vi "Begin.vi"(8 "error in":errorcluster) -> (0 "error out":errorcluster)   [LabVIEW 2020]
doc: "Called before other user functions, this VI is expected to open initial I/O refnums, load in file data, and do all program initialization. Notice that the <B>error out</B> terminal is simply used for data flow. Wiring it to other structures or subVIs ensures that this VI runs first."
uses:
  <vilib>/Rock Robotics/WPI/Encoder/WPI_EncoderType.ctl
  <vilib>/Rock Robotics/SystemInterfaces/DIO/FPGA_DIOChannel.ctl
  <vilib>/Rock Robotics/WPI/ThirdParty/Phoenix-LabVIEW/CANCoder/Controls/CTRE_Phoenix_CANcoder_Configurables.ctl
  <vilib>/Rock Robotics/WPI/ThirdParty/Phoenix-LabVIEW/CANCoder/Controls/CTRE_Phoenix_CANcoder_SensorInitializationStrategy.ctl
  <vilib>/Rock Robotics/WPI/ThirdParty/Phoenix-LabVIEW/CANCoder/Controls/CTRE_Phoenix_CANcoder_AbsoluteSensorRange.ctl
  <vilib>/Rock Robotics/WPI/ThirdParty/Phoenix-LabVIEW/Motor Controller/Controls/CTRE_Phoenix_MotorControl_VelocityMeasurementPeriod.ctl
  <vilib>/Rock Robotics/WPI/ThirdParty/Phoenix-LabVIEW/CANCoder/Controls/CTRE_Phoenix_CANcoder_SensorTimeBase.ctl
  <vilib>/Rock Robotics/WPI/DriverStation/WPI_DriverStationRobotMode2.ctl
  <vilib>/Rock Robotics/WPI/Joystick/WPI_JoystickDeviceEnum.ctl
  <vilib>/Rock Robotics/WPI/ThirdParty/REV Robotics/REVLib/Typedef/Spark MAX Motor Type.ctl
  <vilib>/Rock Robotics/WPI/ThirdParty/REV Robotics/REVLib/Typedef/Spark MAX Idle Mode.ctl
  <vilib>/Rock Robotics/WPI/SafetyOutput/WPI_SafetyOutputConfigMenu.ctl
  <vilib>/Rock Robotics/WPI/Solenoid/WPI_SolenoidChannel.ctl
  <vilib>/Rock Robotics/SystemInterfaces/DIO/FPGA_DIOPWMChannel.ctl
  Robot Global Data.vi
  <vilib>/Rock Robotics/Network Tables/NT Write String Array.vi
  <vilib>/Rock Robotics/WPI/Switch/WPI_SwitchOpenLimit.vi
  <vilib>/Rock Robotics/WPI/RobotDrive/WPI_RobotDriveOpen4MotorWithExistingMotors.vi
  <vilib>/Rock Robotics/WPI/Counter/WPI_CounterDigitalInputToDigitalSource.vi
  <vilib>/Rock Robotics/WPI/Solenoid/WPI_SolenoidOpenDouble.vi
  <vilib>/Rock Robotics/WPI/ThirdParty/Phoenix-LabVIEW/CANCoder/Set/CTRE_Phoenix_CANcoder_SetPosition.vi
panel:
  in  "CANcoder Configurables":T1={"Sensor Initialization Strategy"=enum."Boot To Zero", "Absolute Sensor Range"=enum."Unsigned [0 to 360)", "Velocity Measurement Period"=100, "Velocity Measurement Window"=64, "Magnet Offset (Degrees)"=0.0, "Sensor Direction"=FALSE, "Sensor Coefficient"=0.087890625, "Unit String"="deg", "Sensor Time Base"=enum."PerMinute"} {"Velocity Measurement Period" items=["Period_1ms"=1, "Period_2ms"=2, "Period_5ms"=5, "Period_10ms"=10, "Period_20ms"=20, "Period_25ms"=25, "Period_50ms"=50, "Period_100ms"=100]; "Sensor Coefficient" format="%#_9g"}
  in  "A Channel 2":T6=enum."DIO 2"
  in  "B Channel 2":T6=enum."DIO 3"
  in  "Invert Direction 2":bool
  in  "Decoding Type 2":T7=enum."4x"
  in  "DistancePerCount (Deg) 2":dbl=2.0
  in  "Minimum Rate 2":dbl=20.0
  in  "Number Samples to Average 2":u8=1
  in  "A Channel":T6
  in  "B Channel":T6=enum."DIO 1"
  in  "Invert Direction":bool
  in  "Decoding Type":T7=enum."4x"
  in  "DistancePerCount (Deg)":dbl=2.0
  in  "Minimum Rate":dbl=20.0
  in  "Number Samples to Average":u8=1
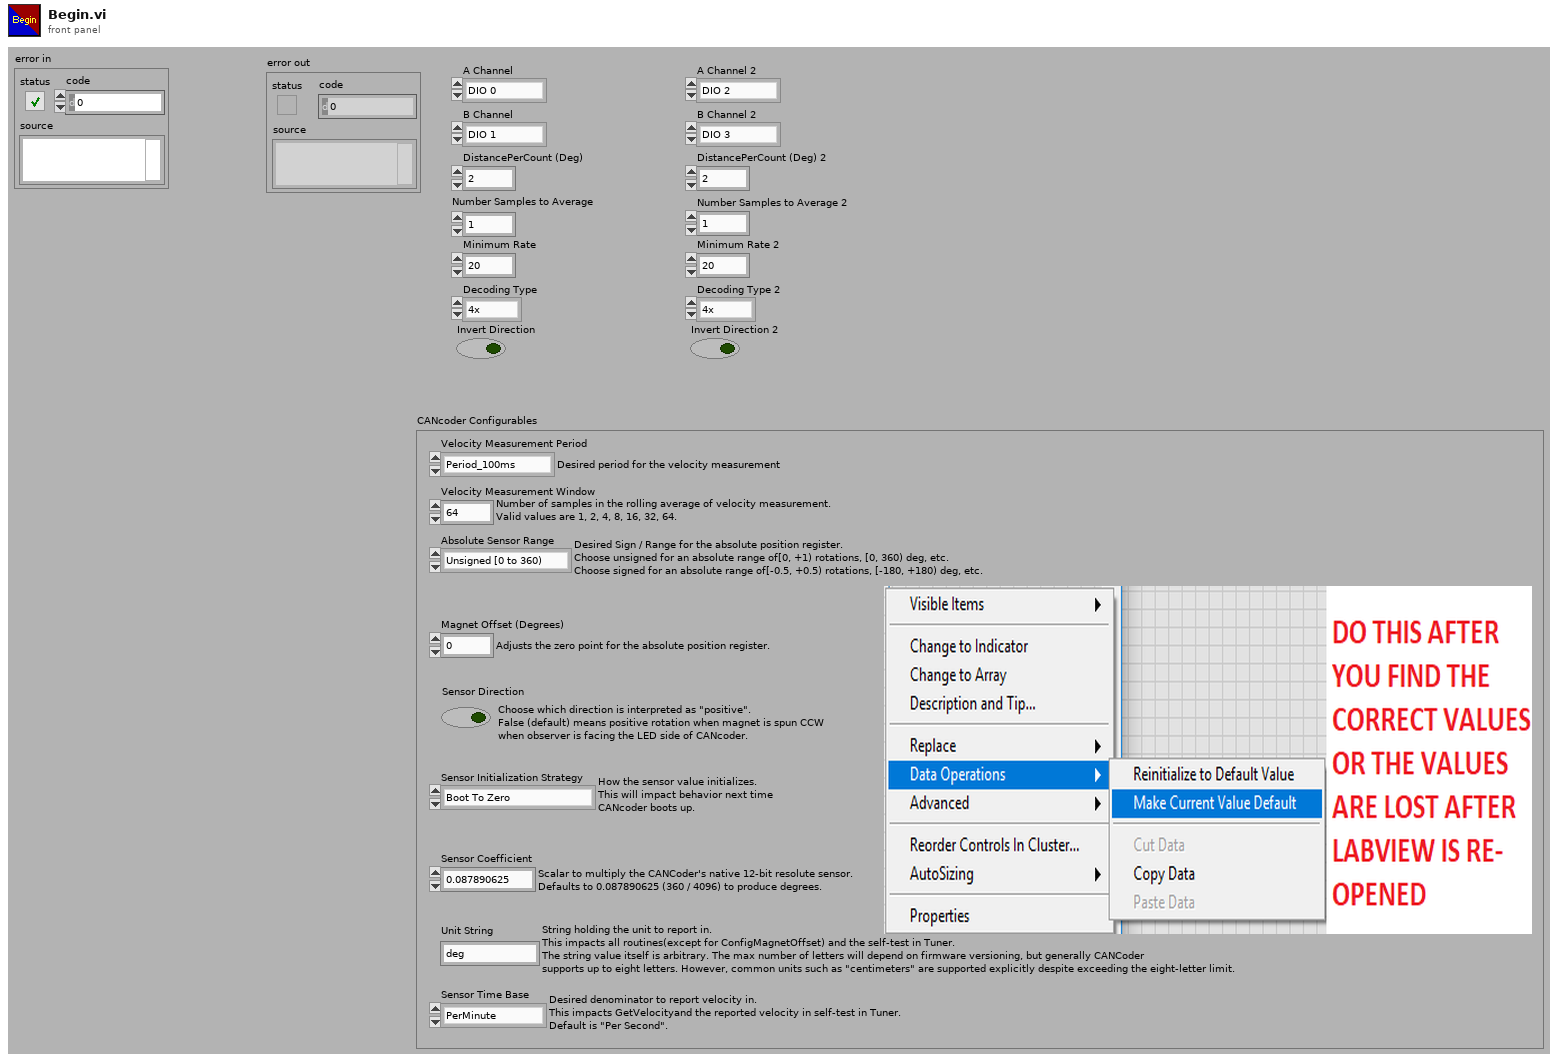
[diagram p1: front panel]
types:
  T1 = typedef "CTRE_Phoenix_CANcoder_Configurables.ctl" = cluster{"Sensor Initialization Strategy":T2, "Absolute Sensor Range":T3, "Velocity Measurement Period":T4, "Velocity Measurement Window":i32, "Magnet Offset (Degrees)":dbl, "Sensor Direction":bool, "Sensor Coefficient":dbl, "Unit String":string, "Sensor Time Base":T5}
  T2 = typedef "CTRE_Phoenix_CANcoder_SensorInitializationStrategy.ctl" = enum16{"Boot To Zero", "Boot To Absolute Position"}
  T3 = typedef "CTRE_Phoenix_CANcoder_AbsoluteSensorRange.ctl" = enum16{"Unsigned [0 to 360)", "Signed [-180 to +180)"}
  T4 = typedef "CTRE_Phoenix_MotorControl_VelocityMeasurementPeriod.ctl" = u16
  T5 = typedef "CTRE_Phoenix_CANcoder_SensorTimeBase.ctl" = enum16{"Per100Ms_Legacy", "PerSecond", "PerMinute"}
  T6 = typedef "FPGA_DIOChannel.ctl" = enum8{"DIO 0", "DIO 1", "DIO 2", "DIO 3", "DIO 4", "DIO 5", "DIO 6", "DIO 7", "DIO 8", "DIO 9", "DIO MXP 0", "DIO MXP 1", "DIO MXP 2", "DIO MXP 3", "DIO MXP 4", "DIO MXP 5", "DIO MXP 6", "DIO MXP 7", "DIO MXP 8", "DIO MXP 9", "DIO MXP 10", "DIO MXP 11", "DIO MXP 12", "DIO MXP 13", "DIO MXP 14", "DIO MXP 15", "SPI Port CS1", "SPI Port CS2", "SPI Port CS3", "SPI Port MISO", "SPI Port MOSI", "Invalid"}
  T7 = typedef "WPI_EncoderType.ctl" = enum16{"1x", "2x", "4x"}
  T8 = typedef "FPGA_DIOPWMChannel.ctl" = enum8{"PWM 0", "PWM 1", "PWM 2", "PWM 3", "PWM 4", "PWM 5", "PWM 6", "PWM 7", "PWM 8", "PWM 9", "PWM MXP 0", "PWM MXP 1", "PWM MXP 2", "PWM MXP 3", "PWM MXP 4", "PWM MXP 5", "PWM MXP 6", "PWM MXP 7", "PWM MXP 8", "PWM MXP 9", "Invalid"}
  T9 = typedef "WPI_SolenoidChannel.ctl" = enum8{"Solenoid 0", "Solenoid 1", "Solenoid 2", "Solenoid 3", "Solenoid 4", "Solenoid 5", "Solenoid 6", "Solenoid 7", "Solenoid 8", "Solenoid 9", "Solenoid 10", "Solenoid 11", "Solenoid 12", "Solenoid 13", "Solenoid 14", "Solenoid 15", "Invalid"}
  T10 = typedef "WPI_SafetyOutputConfigMenu.ctl" = enum16{"Enable", "Disable"}
  T11 = typedef "WPI_JoystickDeviceEnum.ctl" = enum16{"USB 0", "USB 1", "USB 2", "USB 3", "USB 4", "USB 5"}
  T12 = typedef "Spark MAX Idle Mode.ctl" = enum16{"Coast", "Brake"}
  T13 = typedef "Spark MAX Motor Type.ctl" = enum16{"Brushed", "Brushless"}
  T14 = typedef "WPI_DriverStationRobotMode2.ctl" = enum16{"Autonomous Disabled", "Autonomous Enabled", "Teleop Disabled", "Teleop Enabled", "Disconnected", "Finish", "Test Disabled", "Test Enabled", "Emergency Stopped"}
  T15 = typedef "WPI_MotorControlDeviceRef.ctl" = cluster{"DeviceStatus":errorcluster, "Type":T16, "PWM":cluster{"PWM Channel":T8, "DeadBand":T17}, "CAN":cluster{"Device Number":u8, "SetOutput VI Ref":variant, "GetOutput VI Ref":variant, "Enable VI Ref":variant, "Disable VI Ref":variant, "Data":variant}, "Invert":bool, "DIO PWM":cluster{"PWM \"Enable\" Channel":T8, "DIOChannel":T6, "PWM Rate":dbl}}
  T16 = typedef "WPI_MotorControlType.ctl" = enum16{"PWM", "CAN", "DIO PWM"}
  T17 = typedef "WPI_PWMDeadband.ctl" = cluster{"Name":string, "maxPositivePwm":i32, "minPositivePwm":i32, "centerPwm":i32, "maxNegativePwm":i32, "minNegativePwm":i32, "angularRange":u16}
  T18 = typedef "WPI_JoystickDevRef.ctl" = cluster{"Device":T11}
  T19 = typedef "WPI_RobotDriveDevRef.ctl" = cluster{"DevStatus":errorcluster, "Motors[]":T15[], "Square Inputs":bool, "Max Output":dbl}
  T20 = typedef "CTRE_Phoenix_CANcoder_DeviceRef.ctl" = cluster{"DeviceStatus":errorcluster, "Device Number":u8, "Handle":u64, "UsageFrame":u32, "Library Path":path}
  T21 = typedef "WPI_DigitalInputDevRef.ctl" = cluster{"DevStatus":errorcluster, "DIO Channel":T6}
  T22 = typedef "FPGA_CounterEncoderSourceConvertionLVSourceType.ctl" = cluster{"DevStatus":errorcluster, "AnalogTriggerMode?":bool, "DigitalMode":cluster{"DIO Channel":T23}, "AnalogTriggerMode":cluster{"AnalogTriggerIndex":T24, "OutputType":T25}}
  T23 = typedef "FPGA_DIODigitalSourceChannel.ctl" = enum8{"DIO 0", "DIO 1", "DIO 2", "DIO 3", "DIO 4", "DIO 5", "DIO 6", "DIO 7", "DIO 8", "DIO 9", "DIO MXP 0", "DIO MXP 1", "DIO MXP 2", "DIO MXP 3", "DIO MXP 4", "DIO MXP 5", "DIO MXP 6", "DIO MXP 7", "DIO MXP 8", "DIO MXP 9", "DIO MXP 10", "DIO MXP 11", "DIO MXP 12", "DIO MXP 13", "DIO MXP 14", "DIO MXP 15", "SPI Port CS1", "SPI Port CS2", "SPI Port CS3", "SPI Port MISO", "SPI Port MOSI", "Disabled"}
  T24 = typedef "FPGA_AnalogTriggerIndex.ctl" = enum8{"Trig 0", "Trig 1", "Trig 2", "Trig 3", "Trig 4", "Trig 5", "Trig 6", "Trig 7", "Invalid"}
  T25 = typedef "FPGA_AnalogTriggerOutType.ctl" = enum16{"InWindow", "TriggerState", "Rising", "Falling"}
  T26 = typedef "WPI_ServoDeviceRef.ctl" = cluster{"DeviceStatus":errorcluster, "PWM Channel":T8, "DeadBand":T17}
  T27 = typedef "WPI_EncoderDevRef.ctl" = cluster{"DevStatus":errorcluster, "EncoderIndex":T28, "CounterIndex":T29, "DistancePerCount":dbl, "Decoding Type":T7}
  T28 = typedef "FPGA_EncoderIdx.ctl" = enum8{"Enc 0", "Enc 1", "Enc 2", "Enc 3", "Enc 4", "Enc 5", "Enc 6", "Enc 7", "Invalid"}
  T29 = typedef "FPGA_CounterCtrSystemIndex.ctl" = enum8{"Ctr 0", "Ctr 1", "Ctr 2", "Ctr 3", "Ctr 4", "Ctr 5", "Ctr 6", "Ctr 7", "Invalid"}
  T30 = typedef "WPI_SwitchDevRef.ctl" = cluster{"DevStatus":errorcluster, "DIO Channel":T6, "CntIndex":T29, "Normally Closed":bool}
  T31 = typedef "WPI_SolenoidDevRef.ctl" = cluster{"DevStatus":errorcluster, "Pneumatics Control Module":u8, "Forward Solenoid Channel":T9, "Reverse Solenoid Channel":T9}
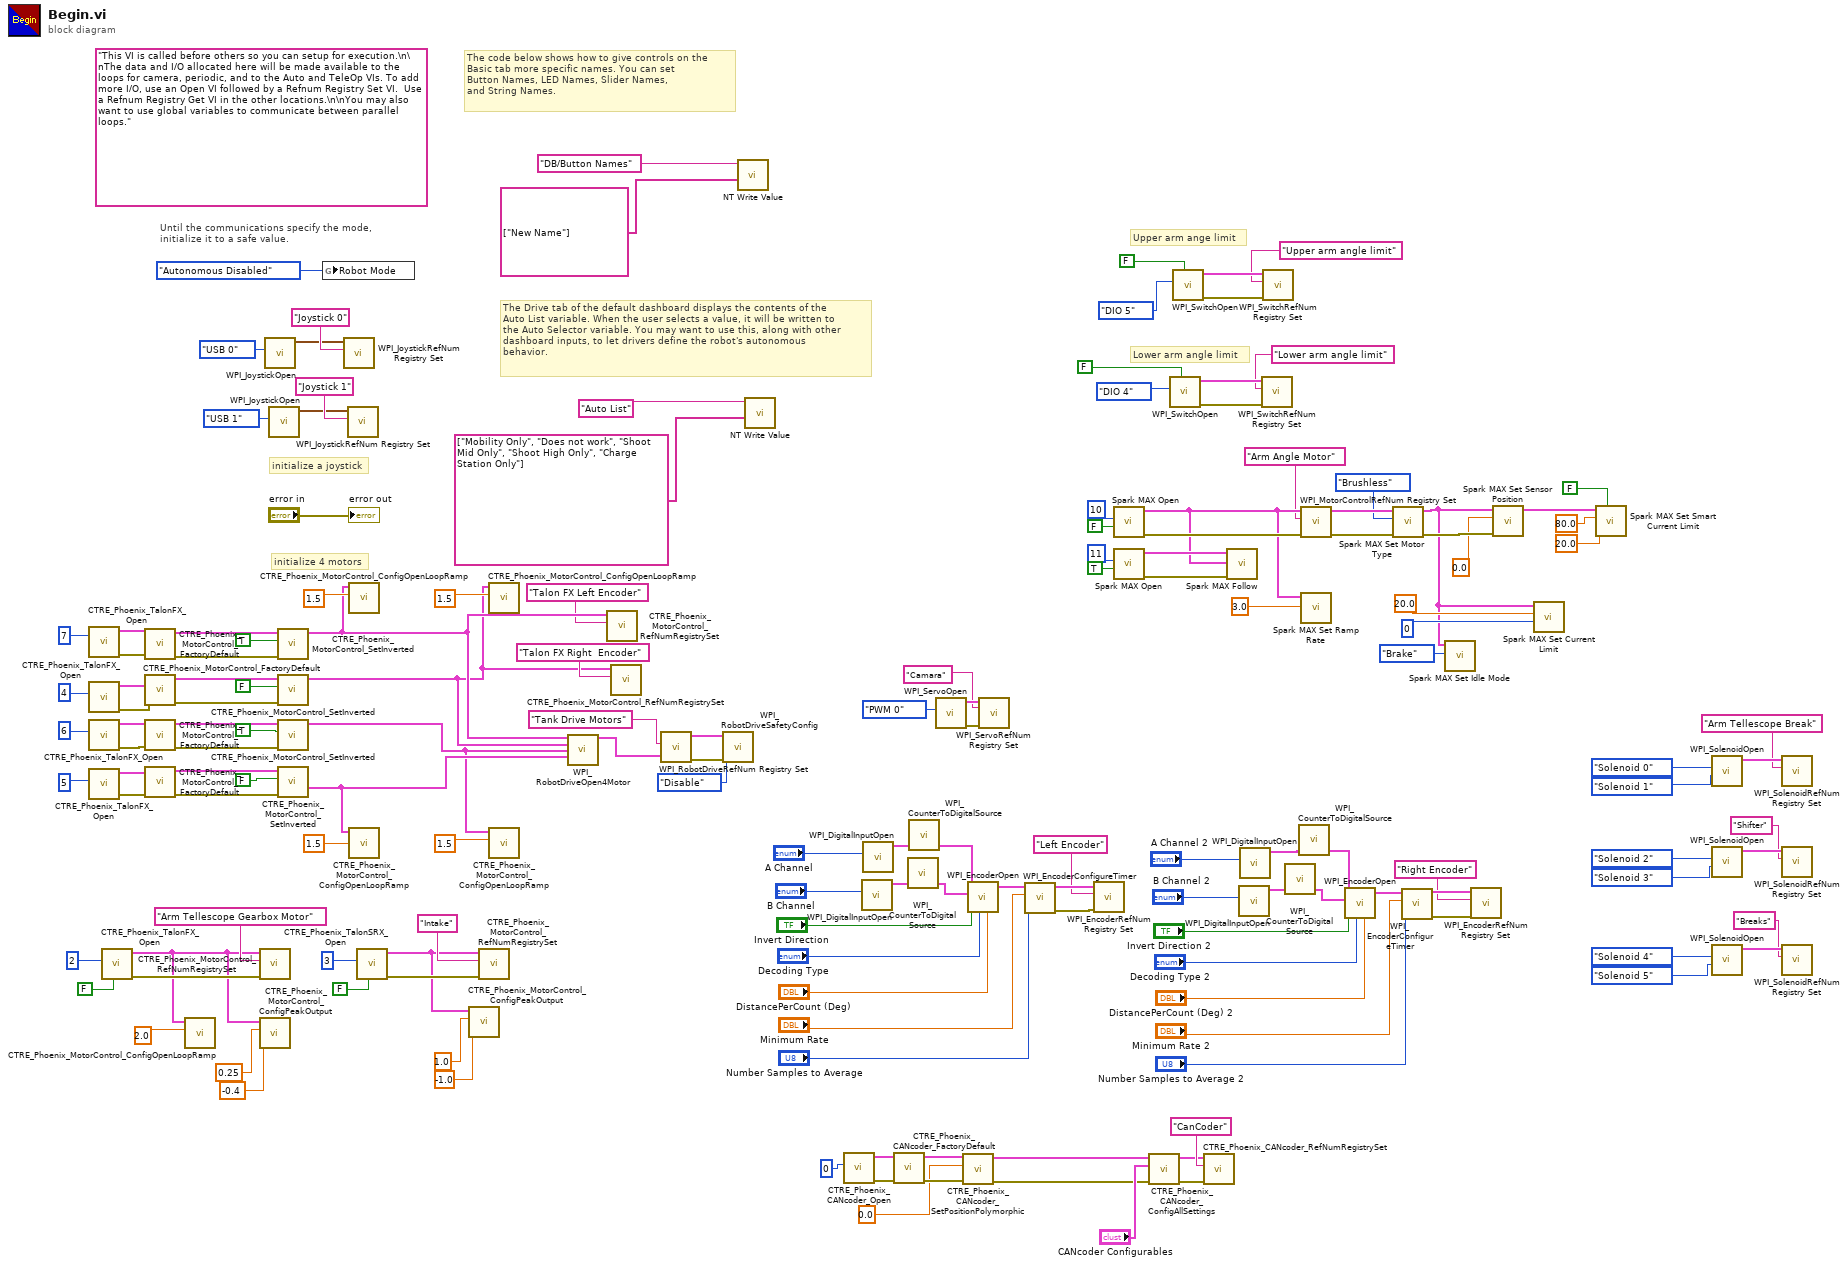
[diagram p0: block diagram]
diagram:
  (unwired) "This VI is called before others so you can setup for execution.\n\nThe data and I/O allocated here will be made available to the loops for camera, periodic, and to the Auto and TeleOp VIs. To add more I/O, use an Open VI followed by a Refnum Registry Set VI.  Use a Refnum Registry Get VI in the other locations.\n\nYou may also want to use global variables to communicate between parallel loops."
  # "Lower arm angle limit"
  # "Upper arm ange limit"
  # "The Drive tab of the default dashboard displays the contents of the\nAuto List variable. When the user selects a value, it will be written to\nthe Auto Selector variable. You may want to use this, along with other\ndashboard inputs, to let drivers define the robot's autonomous\nbehavior."
  # "The code below shows how to give controls on the\nBasic tab more specific names. You can set\nButton Names, LED Names, Slider Names,\nand String Names."
  # "initialize a joystick"
  # "Until the communications specify the mode,\ninitialize it to a safe value."
  # "initialize 4 motors"
  n1 = call <vilib>:"CTRE_Phoenix_TalonFX_Open.vi"("Device Number"=u8 7) -> ("error out"=w92:errorcluster, "PhoenixMotorControlDevRef"=w90:T15)  [unwired: 9 in]
  n2 = call <vilib>:"CTRE_Phoenix_TalonFX_Open.vi"("Device Number"=u8 4) -> ("error out"=w94:errorcluster, "PhoenixMotorControlDevRef"=w95:T15)  [unwired: 9 in]
  n3 = call <vilib>:"CTRE_Phoenix_TalonFX_Open.vi"("Device Number"=u8 6) -> ("error out"=w98:errorcluster, "PhoenixMotorControlDevRef"=w99:T15)  [unwired: 9 in]
  n4 = call <vilib>:"CTRE_Phoenix_TalonFX_Open.vi"("Device Number"=u8 5) -> ("error out"=w80:errorcluster, "PhoenixMotorControlDevRef"=w100:T15)  [unwired: 9 in]
  n5 = call <vilib>:"CTRE_Phoenix_TalonFX_Open.vi"("Invert"=FALSE, "Device Number"=u8 2) -> ("error out"=w37:errorcluster, "PhoenixMotorControlDevRef"=w33:T15)  [unwired: 8 in]
  n6 = call <vilib>:"CTRE_Phoenix_MotorControl_FactoryDefault.vi"("error in"=w92, "PhoenixMotorControlDevRef"=w90) -> ("error out"=w91:errorcluster, "PhoenixMotorControlDevRef"=w89:T15)  [unwired: 8 in]
  n7 = call <vilib>:"CTRE_Phoenix_MotorControl_FactoryDefault.vi"("error in"=w94, "PhoenixMotorControlDevRef"=w95) -> ("error out"=w110:errorcluster, "PhoenixMotorControlDevRef"=w111:T15)  [unwired: 8 in]
  n8 = call <vilib>:"CTRE_Phoenix_MotorControl_FactoryDefault.vi"("error in"=w98, "PhoenixMotorControlDevRef"=w99) -> ("error out"=w112:errorcluster, "PhoenixMotorControlDevRef"=w113:T15)  [unwired: 8 in]
  n9 = call <vilib>:"CTRE_Phoenix_MotorControl_FactoryDefault.vi"("error in"=w80, "PhoenixMotorControlDevRef"=w100) -> ("error out"=w108:errorcluster, "PhoenixMotorControlDevRef"=w109:T15)  [unwired: 8 in]
  n10 = call <vilib>:"CTRE_Phoenix_MotorControl_ConfigOpenLoopRamp.vi"("secondsFromNeutralToFull"=2.0, "PhoenixMotorControlDevRef"=w33) -> ()  [unwired: 8 in, 2 out]
  n11 = call <vilib>:"CTRE_Phoenix_MotorControl_RefNumRegistrySet.vi"("error in (no error)"=w37, "refnum name"="Arm Tellescope Gearbox Motor", "PhoenixMotorControlDevRef"=w33) -> ()  [unwired: 7 in, 2 out]
  n12 = call <vilib>:"CTRE_Phoenix_MotorControl_ConfigPeakOutput.vi"("Reverse Peak Percent Output"=-0.4, "Forward Peak Percent Output"=0.25, "PhoenixMotorControlDevRef"=w33) -> ()  [unwired: 7 in, 2 out]
  n13 = call <vilib>:"WPI_JoystickOpen.vi"("JoystickDevice"=WPI_JoystickDeviceEnum."USB 0") -> ("JoystickDevRef"=w155:T18)  [unwired: 10 in]
  n14 = call <vilib>:"WPI_JoystickOpen.vi"("JoystickDevice"=WPI_JoystickDeviceEnum."USB 1") -> ("JoystickDevRef"=w115:T18)  [unwired: 10 in]
  n15 = call <vilib>:"CTRE_Phoenix_MotorControl_SetInverted.vi"("error in (no error)"=w91, "Invert?"=TRUE, "PhoenixMotorControlDevRef"=w89) -> ("PhoenixMotorControlDevRef"=w9:T15)  [unwired: 7 in, 1 out]
  n16 = call <vilib>:"CTRE_Phoenix_MotorControl_SetInverted.vi"("error in (no error)"=w110, "Invert?"=FALSE, "PhoenixMotorControlDevRef"=w111) -> ("PhoenixMotorControlDevRef"=w6:T15)  [unwired: 7 in, 1 out]
  n17 = call <vilib>:"CTRE_Phoenix_MotorControl_SetInverted.vi"("error in (no error)"=w112, "Invert?"=TRUE, "PhoenixMotorControlDevRef"=w113) -> ("PhoenixMotorControlDevRef"=w81:T15)  [unwired: 7 in, 1 out]
  n18 = call <vilib>:"CTRE_Phoenix_MotorControl_SetInverted.vi"("error in (no error)"=w108, "Invert?"=FALSE, "PhoenixMotorControlDevRef"=w109) -> ("PhoenixMotorControlDevRef"=w82:T15)  [unwired: 7 in, 1 out]
  n19 = global write "Robot Global Data.vi" "Robot Mode"(WPI_DriverStationRobotMode2."Autonomous Disabled" ("Robot Mode")) -> ()
  n20 = call <vilib>:"WPI_JoystickRefNum Registry Set.vi"("refnum name"="Joystick 0", "JoystickDevRef"=w155) -> ()  [unwired: 8 in, 2 out]
  n21 = call <vilib>:"WPI_JoystickRefNum Registry Set.vi"("refnum name"="Joystick 1", "JoystickDevRef"=w115) -> ()  [unwired: 8 in, 2 out]
  n22 = call <vilib>:"CTRE_Phoenix_MotorControl_ConfigOpenLoopRamp.vi"("secondsFromNeutralToFull"=1.5, "PhoenixMotorControlDevRef"=w9) -> ()  [unwired: 8 in, 2 out]
  n23 = call <vilib>:"CTRE_Phoenix_MotorControl_ConfigOpenLoopRamp.vi"("secondsFromNeutralToFull"=1.5, "PhoenixMotorControlDevRef"=w82) -> ()  [unwired: 8 in, 2 out]
  n24 = call <vilib>:"CTRE_Phoenix_TalonSRX_Open.vi"("Invert"=FALSE, "Device Number"=u8 3) -> ("error out"=w28:errorcluster, "PhoenixMotorControlDevRef"=w17:T15)  [unwired: 8 in]
  n25 = call <vilib>:"CTRE_Phoenix_MotorControl_ConfigPeakOutput.vi"("Reverse Peak Percent Output"=-1.0, "Forward Peak Percent Output"=1.0, "PhoenixMotorControlDevRef"=w17) -> ()  [unwired: 7 in, 2 out]
  n26 = call <vilib>:"CTRE_Phoenix_MotorControl_RefNumRegistrySet.vi"("error in (no error)"=w28, "refnum name"="Intake", "PhoenixMotorControlDevRef"=w17) -> ()  [unwired: 7 in, 2 out]
  n27 = call <vilib>:"CTRE_Phoenix_MotorControl_ConfigOpenLoopRamp.vi"("secondsFromNeutralToFull"=1.5, "PhoenixMotorControlDevRef"=w6) -> ()  [unwired: 8 in, 2 out]
  n28 = call <vilib>:"CTRE_Phoenix_MotorControl_ConfigOpenLoopRamp.vi"("secondsFromNeutralToFull"=1.5, "PhoenixMotorControlDevRef"=w81) -> ()  [unwired: 8 in, 2 out]
  n29 = call-poly <vilib>:"WPI_RobotDriveOpen4Motor.vi"("Rear Left Motor Dev Ref"=w9, "Rear Right Motor Dev Ref"=w6, "Front Left Motor Dev Ref"=w81, "Front Right Motor Dev Ref"=w82) -> ("RobotDriveDevRef"=w104:T19)  [unwired: 10 in, 1 out]
  n30 = call <vilib>:"CTRE_Phoenix_MotorControl_RefNumRegistrySet.vi"("refnum name"="Talon FX Left Encoder", "PhoenixMotorControlDevRef"=w9) -> ()  [unwired: 8 in, 2 out]
  n31 = call <vilib>:"CTRE_Phoenix_MotorControl_RefNumRegistrySet.vi"("refnum name"="Talon FX Right  Encoder", "PhoenixMotorControlDevRef"=w6) -> ()  [unwired: 8 in, 2 out]
  n32 = call <vilib>:"WPI_RobotDriveRefNum Registry Set.vi"("refnum name"="Tank Drive Motors", "RobotDriveDevRef"=w104) -> ("error out"=w84:errorcluster, "RobotDriveDevRef"=w86:T19)  [unwired: 8 in]
  n33 = call <vilib>:"WPI_RobotDriveSafetyConfig.vi"("error in (no error)"=w84, "mode"=WPI_SafetyOutputConfigMenu."Disable", "RobotDriveDevRef"=w86) -> ()  [unwired: 7 in, 2 out]
  n34 = call-poly <vilib>:"NT Write Value.vi"("value"=string[] ["New Name"], "name"="DB/Button Names" ("Name")) -> ()  [unwired: 9 in, 1 out]
  n35 = call-poly <vilib>:"NT Write Value.vi"("value"=string[] ["Mobility Only", "Does not work", "Shoot Mid Only", "Shoot High Only", "Charge Station Only"] ("String Array"), "name"="Auto List" ("Name")) -> ()  [unwired: 9 in, 1 out]
  n36 = call <vilib>:"CTRE_Phoenix_CANcoder_Open.vi"("Device Number"=u8 0) -> ("error out"=w25:errorcluster, "CTRE_CANcoder_DeviceRef"=w26:T20)  [unwired: 9 in]
  n37 = call <vilib>:"WPI_DigitalInputOpen.vi"("DIO Channel"="B Channel") -> ("DigitalInputDevRef"=w71:T21)  [unwired: 1 in, 9 out]
  n38 = call <vilib>:"WPI_DigitalInputOpen.vi"("DIO Channel"="A Channel") -> ("DigitalInputDevRef"=w72:T21)  [unwired: 1 in, 9 out]
  n39 = call <vilib>:"CTRE_Phoenix_CANcoder_FactoryDefault.vi"("error in"=w25, "CTRE_CANcoder_DeviceRef"=w26) -> ("error out"=w15:errorcluster, "CTRE_CANcoder_DeviceRef"=w16:T20)  [unwired: 8 in]
  n40 = call-poly <vilib>:"WPI_CounterToDigitalSource.vi"("DigitalInputDevRef"=w71) -> ("Digital Source"=w67:T22)  [unwired: 6 out]
  n41 = call-poly <vilib>:"WPI_CounterToDigitalSource.vi"("DigitalInputDevRef"=w72) -> ("Digital Source"=w68:T22)  [unwired: 6 out]
  n42 = call <vilib>:"WPI_ServoOpen.vi"("PWM Channel"=FPGA_DIOPWMChannel."PWM 0") -> ("error out"=w4:errorcluster, "ServoDeviceRef"=w3:T26)  [unwired: 9 in]
  n43 = call-poly <vilib>:"CTRE_Phoenix_CANcoder_SetPositionPolymorphic.vi"("error in (no error)"=w15, "Position"=0.0, "CTRE_CANcoder_DeviceRef"=w16) -> ("error out"=w13:errorcluster, "CTRE_CANcoder_DeviceRef"=w14:T20)  [unwired: 7 in]
  n44 = call <vilib>:"WPI_EncoderOpen.vi"("DistancePerCount"="DistancePerCount (Deg)", "Decoding Type"="Decoding Type", "Invert Direction (False)"="Invert Direction", "BSource"=w67, "ASource"=w68) -> ("EncoderDevRef"=w76:T27)  [unwired: 5 in, 1 out]
  n45 = call <vilib>:"WPI_ServoRefNum Registry Set.vi"("error in (no error)"=w4, "refnum name"="Camara", "ServoDeviceRef"=w3) -> ()  [unwired: 7 in, 2 out]
  n46 = call <vilib>:"WPI_EncoderConfigureTimer.vi"("Number Samples to Average"="Number Samples to Average", "Minimum Rate"="Minimum Rate", "EncoderDevRef"=w76) -> ("error out"=w65:errorcluster, "EncoderDevRef"=w66:T27)  [unwired: 7 in]
  n47 = call <vilib>:"WPI_EncoderRefNum Registry Set.vi"("error in (no error)"=w65, "refnum name"="Left Encoder", "EncoderDevRef"=w66) -> ()  [unwired: 7 in, 2 out]
  n48 = call <vilib>:"Spark MAX Open.vi"("Invert"=FALSE, "Device Number"=u8 10) -> ("error out"=w135:errorcluster, "MotorControlDeviceRef"=w134:T15)  [unwired: 8 in]
  n49 = call <vilib>:"Spark MAX Open.vi"("Invert"=TRUE, "Device Number"=u8 11) -> ("error out"=w144:errorcluster, "MotorControlDeviceRef"=w136:T15)  [unwired: 8 in]
  n50 = call <vilib>:"CTRE_Phoenix_CANcoder_ConfigAllSettings.vi"("error in (no error)"=w13, "CANcoder Configurables"="CANcoder Configurables", "CTRE_CANcoder_DeviceRef"=w14) -> ("error out"=w21:errorcluster, "CTRE_CANcoder_DeviceRef"=w22:T20)  [unwired: 7 in]
  n51 = call-poly <vilib>:"WPI_SwitchOpen.vi"("Normally Closed"=FALSE, "DIO Channel"=FPGA_DIOChannel."DIO 4") -> ("error out"=w124:errorcluster, "SwitchDevRef"=w125:T30)  [unwired: 8 in]
  n52 = call-poly <vilib>:"WPI_SwitchOpen.vi"("Normally Closed"=FALSE, "DIO Channel"=FPGA_DIOChannel."DIO 5") -> ("error out"=w123:errorcluster, "SwitchDevRef"=w126:T30)  [unwired: 8 in]
  n53 = call <vilib>:"CTRE_Phoenix_CANcoder_RefNumRegistrySet.vi"("error in (no error)"=w21, "refnum name"="CanCoder", "CTRE_CANcoder_DeviceRef"=w22) -> ()  [unwired: 7 in, 2 out]
  n54 = call <vilib>:"Spark MAX Follow.vi"("error in (no error)"=w144, "Master Controller"=w134, "MotorControlDeviceRef"=w136) -> ()  [unwired: 7 in, 2 out]
  n55 = call <vilib>:"WPI_DigitalInputOpen.vi"("DIO Channel"="B Channel 2") -> ("DigitalInputDevRef"=w57:T21)  [unwired: 1 in, 9 out]
  n56 = call <vilib>:"WPI_DigitalInputOpen.vi"("DIO Channel"="A Channel 2") -> ("DigitalInputDevRef"=w58:T21)  [unwired: 1 in, 9 out]
  n57 = call <vilib>:"WPI_SwitchRefNum Registry Set.vi"("error in (no error)"=w124, "refnum name"="Lower arm angle limit", "SwitchDevRef"=w125) -> ()  [unwired: 7 in, 2 out]
  n58 = call <vilib>:"WPI_SwitchRefNum Registry Set.vi"("error in (no error)"=w123, "refnum name"="Upper arm angle limit", "SwitchDevRef"=w126) -> ()  [unwired: 7 in, 2 out]
  n59 = call-poly <vilib>:"WPI_CounterToDigitalSource.vi"("DigitalInputDevRef"=w57) -> ("Digital Source"=w53:T22)  [unwired: 6 out]
  n60 = call-poly <vilib>:"WPI_CounterToDigitalSource.vi"("DigitalInputDevRef"=w58) -> ("Digital Source"=w54:T22)  [unwired: 6 out]
  n61 = call <vilib>:"WPI_MotorControlRefNum Registry Set.vi"("error in (no error)"=w135, "refnum name"="Arm Angle Motor", "MotorControlDevRef"=w134) -> ("error out"=w131:errorcluster, "MotorControlDevRef"=w145:T15)  [unwired: 7 in]
  n62 = call <vilib>:"Spark MAX Set Ramp Rate.vi"("Seconds from neutral to full (0)"=sgl 3.0, "MotorControlDeviceRef in"=w134) -> ()  [unwired: 8 in, 2 out]
  n63 = call <vilib>:"WPI_EncoderOpen.vi"("DistancePerCount"="DistancePerCount (Deg) 2", "Decoding Type"="Decoding Type 2", "Invert Direction (False)"="Invert Direction 2", "BSource"=w53, "ASource"=w54) -> ("EncoderDevRef"=w62:T27)  [unwired: 5 in, 1 out]
  n64 = call <vilib>:"Spark MAX Set Motor Type.vi"("error in (no error)"=w131, "Motor Type"=Spark_MAX_Motor_Type."Brushless", "MotorControlDevRef"=w145) -> ("error out"=w130:errorcluster, "MotorControlDeviceRef"=w1:T15)  [unwired: 7 in]
  n65 = call <vilib>:"WPI_EncoderConfigureTimer.vi"("Number Samples to Average"="Number Samples to Average 2", "Minimum Rate"="Minimum Rate 2", "EncoderDevRef"=w62) -> ("error out"=w51:errorcluster, "EncoderDevRef"=w52:T27)  [unwired: 7 in]
  n66 = call <vilib>:"Spark MAX Set Idle Mode.vi"("Idle Mode"=Spark_MAX_Idle_Mode."Brake", "MotorControlDeviceRef in"=w1) -> ()  [unwired: 8 in, 2 out]
  n67 = call <vilib>:"WPI_EncoderRefNum Registry Set.vi"("error in (no error)"=w51, "refnum name"="Right Encoder", "EncoderDevRef"=w52) -> ()  [unwired: 7 in, 2 out]
  n68 = call <vilib>:"Spark MAX Set Sensor Position.vi"("error in"=w130, "Position"=0.0, "MotorControlDeviceRef"=w1) -> ("MotorControlDeviceRef"=w128:T15)  [unwired: 7 in, 1 out]
  n69 = call <vilib>:"Spark MAX Set Current Limit.vi"("Limit Duration (0)"=u32 0, "Current Limit A (100)"=sgl 20.0, "MotorControlDeviceRef in"=w1) -> ()  [unwired: 7 in, 2 out]
  n70 = call <vilib>:"Spark MAX Set Smart Current Limit.vi"("Linearized Limit Enabled (F)"=FALSE, "Free Speed Current Limit (20A)"=20.0, "Primay Current Limit (80A)"=80.0, "MotorControlDeviceRef in"=w128) -> ()  [unwired: 6 in, 2 out]
  n71 = call-poly <vilib>:"WPI_SolenoidOpen.vi"("Reverse Solenoid Channel"=WPI_SolenoidChannel."Solenoid 1" ("Forward Solenoid Channel"), "Forward Solenoid Channel"=WPI_SolenoidChannel."Solenoid 0") -> ("SolenoidDevRef"=w46:T31)  [unwired: 8 in, 1 out]
  n72 = call-poly <vilib>:"WPI_SolenoidOpen.vi"("Reverse Solenoid Channel"=WPI_SolenoidChannel."Solenoid 3" ("Forward Solenoid Channel"), "Forward Solenoid Channel"=WPI_SolenoidChannel."Solenoid 2") -> ("SolenoidDevRef"=w47:T31)  [unwired: 8 in, 1 out]
  n73 = call-poly <vilib>:"WPI_SolenoidOpen.vi"("Reverse Solenoid Channel"=WPI_SolenoidChannel."Solenoid 5" ("Forward Solenoid Channel"), "Forward Solenoid Channel"=WPI_SolenoidChannel."Solenoid 4") -> ("SolenoidDevRef"=w41:T31)  [unwired: 8 in, 1 out]
  n74 = call <vilib>:"WPI_SolenoidRefNum Registry Set.vi"("refnum name"="Arm Tellescope Break", "SolenoidDevRef"=w46) -> ()  [unwired: 8 in, 2 out]
  n75 = call <vilib>:"WPI_SolenoidRefNum Registry Set.vi"("refnum name"="Shifter", "SolenoidDevRef"=w47) -> ()  [unwired: 8 in, 2 out]
  n76 = call <vilib>:"WPI_SolenoidRefNum Registry Set.vi"("refnum name"="Breaks", "SolenoidDevRef"=w41) -> ()  [unwired: 8 in, 2 out]
  "error out" <- "error in"
